vi "GEOM_GetWCSOverride_data_mext.vi"(9 "override headers":string[][][](array[string]), 10 "msheaders in":string[][][](array[string])) -> (2 "mheaders out":string[][][](array[string]))   [LabVIEW 2016]
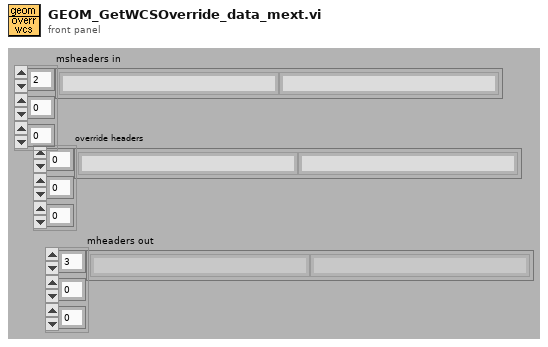
[diagram p1: front panel]
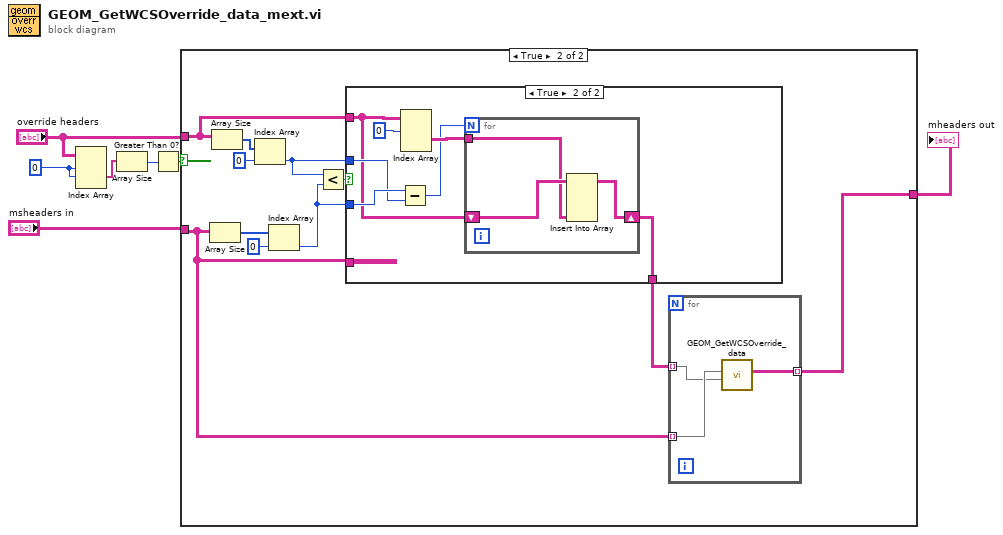
[diagram p0: block diagram]
diagram:
  w1 = 0 ("disabled index (col)")
  n1 = Index Array(array="override headers", index (dim 0)=w1, index (dim 1)=w1) -> (element=w2:string[])  [unwired: 1 in]
  n2 = Array Size(array=w2) -> (size(s)=w7:i32)
  n3 = Greater Than 0?(x=w7) -> (x > 0?=w6:bool)
  n4 = case shown="True" w6 {
    tunnel: "override headers" -> [_ w14]
    tunnel: "msheaders in" -> [w8 w11]
    tunnel: [w8 w12] -> w4
    frame False {
    }
    frame True {
      n5 = Array Size(array=w11) -> (size(s)=w17:i32[])
      n6 = Array Size(array=w14) -> (size(s)=w19:i32[])
      n7 = Index Array(array=w19, index=0) -> (element=w9:i32)
      n8 = Index Array(array=w17, index=0) -> (element=w10:i32)
      n9 = Less?(x=w9, y=w10) -> (x < y?=w15:bool)
      n10 = case shown="True" w15 {
        tunnel: w14 -> [w20 w22]
        tunnel: [w20 w21] -> w13
        tunnel: w11 -> [_ _]
        tunnel: w10 -> [_ w25]
        tunnel: w9 -> [_ w24]
        frame False {
        }
        frame True {
          n11 = Subtract(x=w25, y=w24) -> (x-y=w23:i32)
          n12 = Index Array(array=w22, index (dim 0)=0 ("index (page)")) -> (element=w26:string[][])  [unwired: 2 in]
          n13 = for {
            N: w23 -> [_]
            shift-right: [w28] -> w21
            shift-left: w22 -> [w30]
            tunnel: w26 -> [w29]
            n14 = Insert Into Array(array=w30, new element=w29) -> (w28:string[][][])  [unwired: 3 in]
          }
        }
      }
      n15 = for {
        tunnel: w11 -> [w33] mode=indexing
        tunnel: w13 -> [w32] mode=indexing
        tunnel: [w31] -> w12 mode=indexing
        n16 = call "GEOM_GetWCSOverride_data.vi"("override headers"=w32, "sheaders in"=w33) -> ("sheaders out"=w31:string[][])  [unwired: 9 out]
      }
    }
  }
  "mheaders out" <- w4
